vi "HTTP_Copy_file.vi"(1 "target path":path, 2 "Source Path":path) -> (0 "error out":errorcluster)   [LabVIEW 2010]
doc: "Example of using standard HTTP protocol for recieving a web site (the HTML source)\n\n\nThis example uses the GET command. For general information about the HTTP protocol and other commands go to\nhttp://www.w3.org/Protocols\n\n\nBjornar Svingen\nbjornar.svingen@sintef.no bjornar.svingen@ktv.no"
uses:
  Update_Global.vi
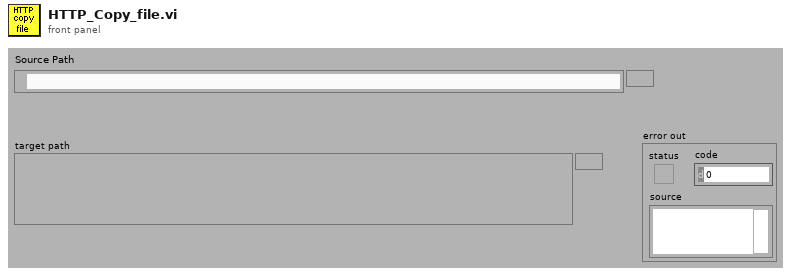
[diagram p1: front panel]
types:
  T1 = enum16{"open", "open or create", "create or replace", "create", "open (read only)"}
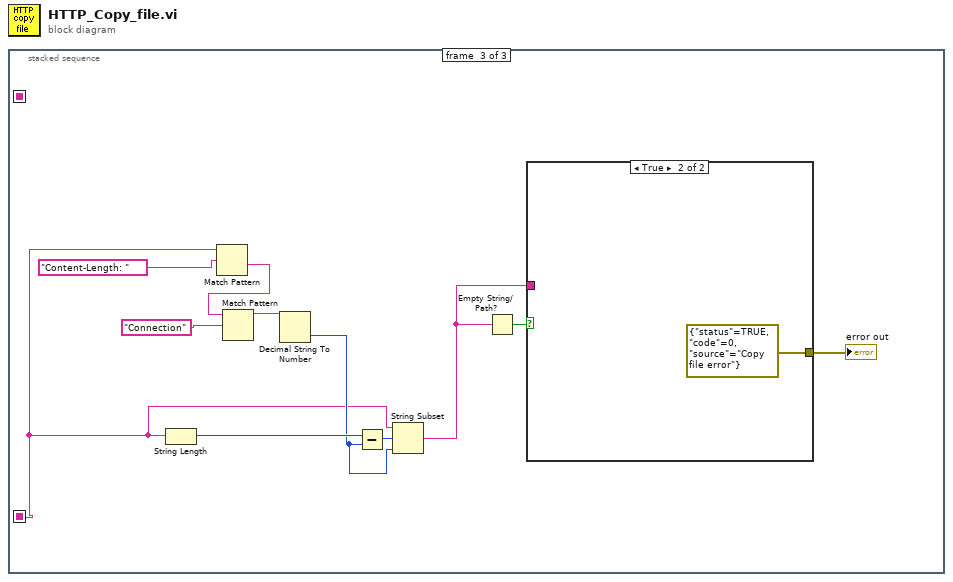
[diagram p0: block diagram]
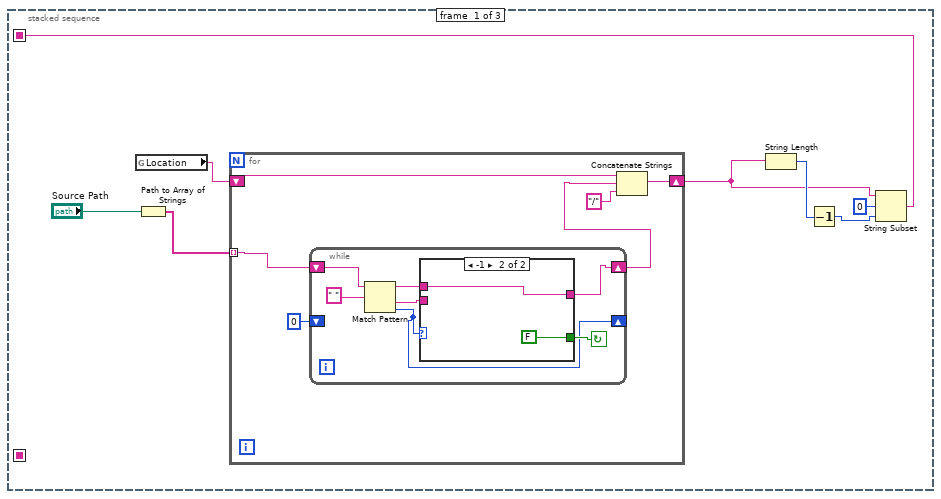
[diagram p2: hidden frame]
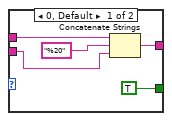
[diagram p3: hidden frame]
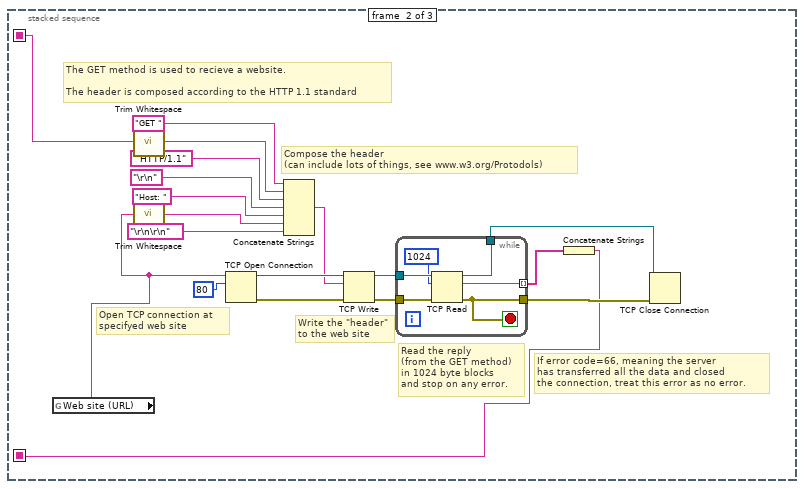
[diagram p4: hidden frame]
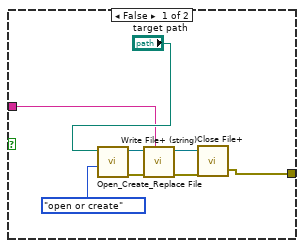
[diagram p5: hidden frame]
diagram:
  n1 = stacked-sequence {
    seq-local: [w2 _ _] -> [_ w31 _]
    seq-local: [_ w29 _] -> [_ _ w56]
    frame #0 {
      n2 = global read "Update_Global.vi" "Location"() -> (w1:string)
      n3 = Path to Array of Strings(0:"Source Path") -> (2:w7:string[])  [unwired: 1 out]
      n4 = for {
        tunnel: w7 -> [w11] mode=indexing
        shift-right: [w12] -> w4
        shift-left: w1 -> [w14]
        n5 = while {
          shift-right: [w16] -> w9
          shift-left: w11 -> [w21]
          shift-right: [w15] -> _
          shift-left: 0 ("offset past match") -> [_]
          stop <- w19 continue-if-true
          n6 = Match Pattern(string=w21, regular expression=" ") -> (before substring=w18:string, after substring=w17:string, offset past match=w15:i32)  [unwired: 2 out]
          n7 = case shown="-1" w15 {
            tunnel: [TRUE FALSE] -> w19
            tunnel: w18 -> [w26 w27]
            tunnel: w17 -> [w24 _]
            tunnel: [w23 w27] -> w16
            frame 0, Default {
              n8 = Concatenate Strings(w26, "%20" ("Replace match with:"), w24) -> (w23:string)
            }
            frame -1 {
            }
          }
        }
        n9 = Concatenate Strings(w14, w9, "/") -> (w12:string)
      }
      n10 = String Length(string=w4) -> (length=w5:i32)
      n11 = Decrement(x=w5) -> (x-1=w3:i32)
      n12 = String Subset(string=w4, offset (0)=0, length (rest)=w3) -> (substring=w2:string)
    }
    frame #1 {
      # "Compose the header\n(can include lots of things, see www.w3.org/Protodols)"
      # "The GET method is used to recieve a website.\n\nThe header is composed according to the HTTP 1.1 standard"
      # "If error code=66, meaning the server\nhas transferred all the data and closed\nthe connection, treat this error as no error."
      # "Read the reply\n(from the GET method)\nin 1024 byte blocks\nand stop on any error."
      # "Write the \"header\"\nto the web site"
      # "Open TCP connection at\nspecifyed web site"
      n13 = global read "Update_Global.vi" "Web site (URL)"() -> (w30:string)
      n14 = call <vilib>:"Trim Whitespace.vi"("string"=w31) -> ("trimmed string"=w38:string)  [unwired: 1 in]
      n15 = call <vilib>:"Trim Whitespace.vi"("string"=w30) -> ("trimmed string"=w34:string)  [unwired: 1 in]
      n16 = TCP Open Connection(address=w30, remote port or service name=u16 80 ("remote port")) -> (connection ID=w46:refnum<k5>, error out=w47:errorcluster)  [unwired: 1 in, 2 out]
      n17 = Concatenate Strings("GET " ("Command"), w38, " HTTP/1.1" ("Command"), "\r\n" ("string"), "Host: " ("Command"), w34, "\r\n\r\n" ("string")) -> (w32:string)
      n18 = TCP Write(connection ID=w46, data in=w32, error in (no error)=w47) -> (connection ID out=w45:refnum<k5>, error out=w44:errorcluster)  [unwired: 2 out]
      n19 = while {
        tunnel: w44 -> [w53]
        tunnel: w45 -> [w52]
        tunnel: [w48] -> w43
        tunnel: [w51] -> w41
        tunnel: [w50] -> w42 mode=indexing
        stop <- w48 stop-if-true
        n20 = TCP Read(connection ID=w52, bytes to read=1024, error in (no error)=w53) -> (connection ID out=w51:refnum<k5>, data out=w50:string, error out=w48:errorcluster)  [unwired: 1 in, 1 out]
      }
      n21 = Concatenate Strings(w42) -> (w29:string)
      n22 = TCP Close Connection(connection ID=w41, error in (no error)=w43) -> ()  [unwired: 3 out]
    }
    frame #2 {
      n23 = String Length(string=w56) -> (length=w59:i32)
      n24 = Match Pattern(string=w56, regular expression="Content-Length: ") -> (after substring=w62:string)  [unwired: 4 out]
      n25 = Match Pattern(string=w62, regular expression="Connection") -> (before substring=w60:string)  [unwired: 4 out]
      n26 = Decimal String To Number(string=w60) -> (number=w58:i32)  [unwired: 3 out]
      n27 = Subtract(x=w59, y=w58) -> (x-y=w57:i32)
      n28 = String Subset(string=w56, offset (0)=w57, length (rest)=w58) -> (substring=w54:string)
      n29 = Empty String/Path?(string/path=w54) -> (empty?=w55:bool)
      n30 = case shown="True" w55 {
        tunnel: [w68 errorcluster {"status"=TRUE, "code"=0, "source"="Copy file error"} ("error out")] -> w64
        tunnel: w54 -> [w65 _]
        frame False {
          n31 = call <vilib>:"Open_Create_Replace File.vi"("function (open:0)"=T1."open or create", "file path"="target path") -> ("error out"=w69:errorcluster, "refnum"=w72:refnum<file>)  [unwired: 4 in, 4 out]
          n32 = call <vilib>:"Write File+ (string).vi"("string"=w65, "error in (no error)"=w69, "refnum"=w72) -> ("error out"=w70:errorcluster, "dup refnum"=w71:refnum<file>)  [unwired: 2 in, 3 out]
          n33 = call <vilib>:"Close File+.vi"("error in (no error)"=w70, "refnum"=w71) -> ("error out"=w68:errorcluster)  [unwired: 5 out]
        }
        frame True {
        }
      }
      "error out" <- w64
    }
  }
